vi "TopLevelControls.vi"() -> ()   [LabVIEW 2016, in "test_ValueSignal.lvlib"]
uses:
  test_ValueSignal.lvlib
  Helper/HelperVI1.vi
  main/apis/Stimulus/ValueSignalByName.vi
  main/apis/Assert/AssertControlValueByName.vi
  <vilib>/addons/_JKI Toolkits/Caraya/classes/Assert/Assert Equal Value_Variant.vi
  <vilib>/addons/_JKI Toolkits/Caraya/classes/Assert/Assert.lvclass
  <vilib>/addons/_JKI Toolkits/Caraya/classes/Test/Test.lvclass
panel:
  out "error out":errorcluster
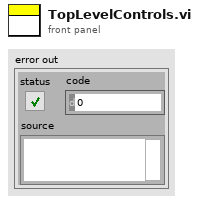
[diagram p1: front panel]
types:
  T1 = cluster{"Numeric_cluster":dbl, "Boolean_cluster":bool, "String_cluster":string}
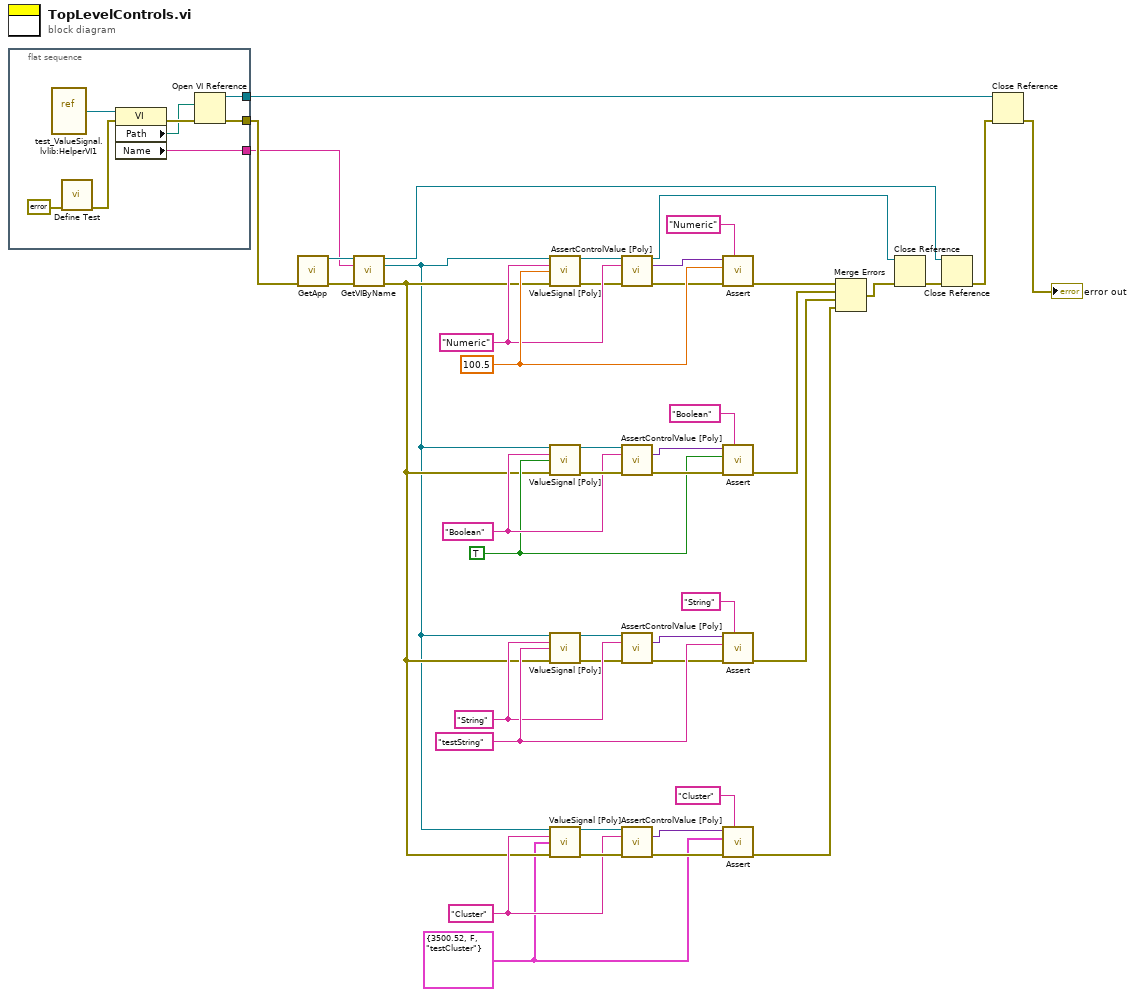
[diagram p0: block diagram]
diagram:
  w2 = T1 {"Numeric_cluster"=3500.52, "Boolean_cluster"=FALSE, "String_cluster"="testCluster"} ("Cluster")
  w7 = "Cluster" ("Class Name")
  w23 = "testString"
  w21 = "String" ("Class Name")
  w26 = TRUE
  w28 = "Boolean" ("Class Name")
  w37 = 100.5
  w35 = "Numeric" ("Class Name")
  n1 = flat-sequence {
    tunnel: [w49] -> w40
    tunnel: [w48] -> w42
    tunnel: [w46] -> w39
    frame #0 {
      n2 = vi-ref "test_ValueSignal.lvlib:HelperVI1.vi"() -> (w51:refnum<vi>)
      n3 = call <vilib>:"Define Test.vi"("error in (no error)"=errorcluster {"status"=FALSE, "code"=0, "source"=""}) -> ("error out"=w52:errorcluster)  [unwired: 10 in]
      n4 = property on="Property Node" class="VI"(reference=w51, error in=w52) -> (error out=w50:errorcluster, "Path"=w47:path, "Name"=w46:string)  [unwired: 1 out]
      n5 = Open VI Reference(vi path=w47, error in (no error)=w50) -> (vi reference=w48:refnum<vi>, error out=w49:errorcluster)  [unwired: 4 in]
    }
  }
  n6 = call "GetApp.vi"("error in (no error)"=w40) -> ("Application Ref"=w41:refnum<vi>, "error out"=w38:errorcluster)  [unwired: 13 in]
  n7 = call "GetVIByName.vi"("Application Ref in"=w41, "VI Name"=w39, "error in (no error)"=w38) -> ("Application Ref out"=w11:refnum<vi>, "VI Reference"=w3:refnum<vi>, "error out"=w4:errorcluster)  [unwired: 10 in]
  n8 = call-poly "ValueSignal [Poly].vi"("VI Reference In"=w3, "Control Name"=w35, "Value (Signaling)"=w37, "error in"=w4) -> ("VI Reference Out"=w36:refnum<vi>, "error out"=w34:errorcluster)  [unwired: 10 in]
  n9 = call-poly "ValueSignal [Poly].vi"("VI Reference In"=w3, "Control Name"=w28, "Value (Signaling)"=w26, "error in"=w4) -> ("VI Reference Out"=w27:refnum<vi>, "error out"=w29:errorcluster)  [unwired: 10 in]
  n10 = call-poly "ValueSignal [Poly].vi"("VI Reference In"=w3, "Control Name"=w21, "Value (Signaling)"=w23, "error in"=w4) -> ("VI Reference Out"=w22:refnum<vi>, "error out"=w20:errorcluster)  [unwired: 10 in]
  n11 = call-poly "ValueSignal [Poly].vi"("VI Reference In"=w3, "Control Name"=w7, "Value (Signaling)"=w2, "error in"=w4) -> ("VI Reference Out"=w6:refnum<vi>, "error out"=w8:errorcluster)  [unwired: 10 in]
  n12 = call-poly "AssertControlValue [Poly].vi"("VI Reference In"=w36, "Control Name"=w35, "error in"=w34) -> ("VI Reference Out"=w13:refnum<vi>, "Value"=w32:variant, "error out"=w33:errorcluster)  [unwired: 10 in]
  n13 = call-poly "AssertControlValue [Poly].vi"("VI Reference In"=w27, "Control Name"=w28, "error in"=w29) -> ("Value"=w31:variant, "error out"=w30:errorcluster)  [unwired: 10 in, 1 out]
  n14 = call-poly "AssertControlValue [Poly].vi"("VI Reference In"=w22, "Control Name"=w21, "error in"=w20) -> ("Value"=w18:variant, "error out"=w19:errorcluster)  [unwired: 10 in, 1 out]
  n15 = call-poly "AssertControlValue [Poly].vi"("VI Reference In"=w6, "Control Name"=w7, "error in"=w8) -> ("Value"=w10:variant, "error out"=w9:errorcluster)  [unwired: 10 in, 1 out]
  n16 = call-poly <vilib>:"Assert.vi"("Label"="Numeric" ("Label (VI Title)"), "error in (no error)"=w33, "Y"=w37, "X"=w32) -> ("error out"=w44:errorcluster)  [unwired: 7 in]
  n17 = call-poly <vilib>:"Assert.vi"("Label"="Boolean" ("Label (VI Title)"), "error in (no error)"=w30, "Y"=w26, "X"=w31) -> ("error out"=w16:errorcluster)  [unwired: 7 in]
  n18 = call-poly <vilib>:"Assert.vi"("Label"="String" ("Label (VI Title)"), "error in (no error)"=w19, "Y"=w23, "X"=w18) -> ("error out"=w15:errorcluster)  [unwired: 7 in]
  n19 = call-poly <vilib>:"Assert.vi"("Label"="Cluster" ("Label (VI Title)"), "error in (no error)"=w9, "Y"=w2, "X"=w10) -> ("error out"=w1:errorcluster)  [unwired: 7 in]
  n20 = Merge Errors(w44, w16, w15, w1) -> (w17:errorcluster)
  n21 = Close Reference(reference=w13, error in (no error)=w17) -> (error out=w14:errorcluster)
  n22 = Close Reference(reference=w11, error in (no error)=w14) -> (error out=w12:errorcluster)
  n23 = Close Reference(reference=w42, error in (no error)=w12) -> (error out=→"error out":errorcluster)
